vi "MENU.vi"() -> ()   [LabVIEW 2019]
panel:
  in  "Tab Control":T1(tab)
  out "DAC 2":dbl
  out "DAC 1":dbl
  in  "ADC 1 control":dbl
  out "ADC 1":dbl(knob) caption="Gauge" scale=0.0..10.0
  in  "DAC 1":dbl(knob) caption="Gauge" scale=0.0..10.0
  out "DI7":bool
  out "DI8":bool
  out "DI9":bool
  out "DI10":bool
  in  "DI7":bool
  in  "DI8":bool
  in  "DI9":bool
  in  "DI10":bool
  in  "DI11":bool
  in  "DI12":bool
  in  "DI13":bool
  out "DI11":bool
  out "DI12":bool
  out "DI13":bool
  in  "DO2 2":bool
  in  "DO3 2":bool
  in  "DO4 2":bool
  out "DO2":bool
  out "DO3":bool
  out "DO4":bool
  in  "DO5 2":bool
  in  "DO6 2":bool
  out "DO5":bool
  out "DO6":bool
  in  "DAC 2":dbl(knob) caption="Gauge" scale=0.0..10.0
  in  "PRODUCCION":bool
  in  "MANUAL":bool
  in  "I/O´S":bool
  in  "ESTADISTICAS":bool
  in  "PRINCIPAL":bool
  in  "stop":bool
  # "BIENVENIDO A LA MAQUINA MKI"
  # "SISTEMA DE PRODUCCIÓN"
  # "ESTADISTICAS DE PRODUCCIÓN"
  # "MONITOR DE ENTRAD Y SALIDAS"
  # "SISTEMA DE CONTROL MANUAL"
  # "ANALOGICO"
  # "SALIDAS"
  # "ENTRADAS"
  # "BYPASS"
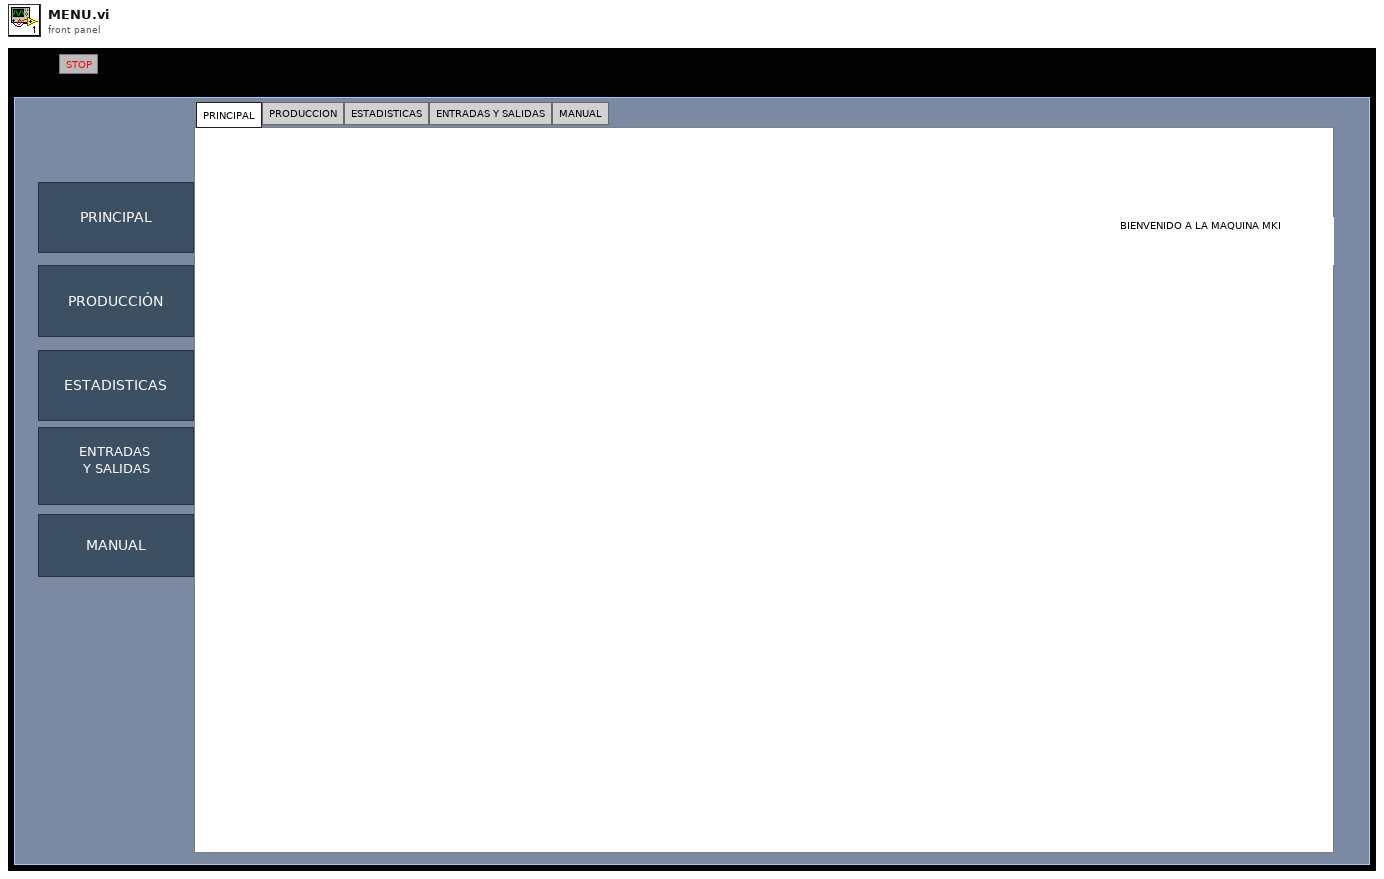
[diagram p1: front panel]
types:
  T1 = enum32{"PRINCIPAL", "PRODUCCION", "ESTADISTICAS", "ENTRADAS Y SALIDAS", "MANUAL"}
  T2 = enum32{"PRINCIPAL", "PPRODUCCION", "ESTADISTICAS", "ENTRADAS Y SALIDAS", "MANUAL"}
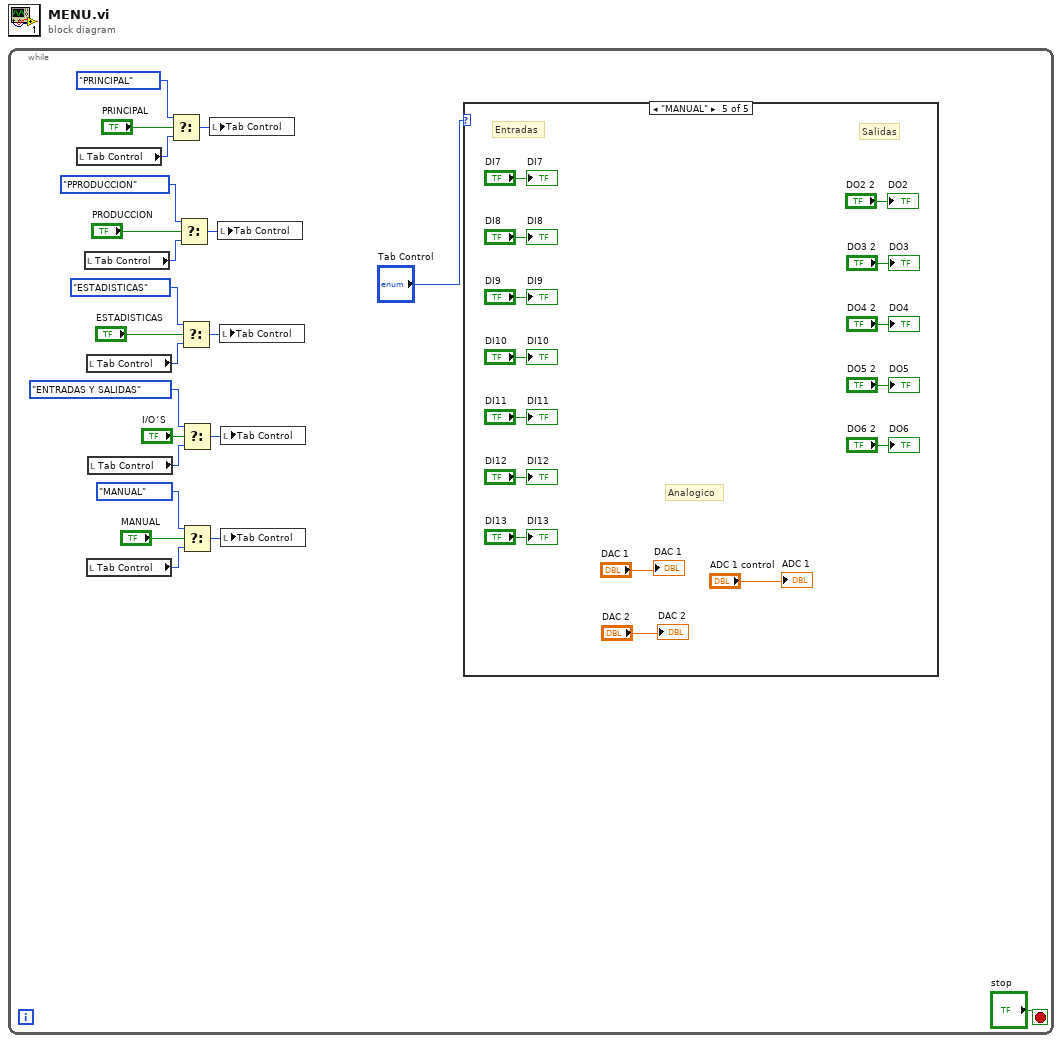
[diagram p0: block diagram]
diagram:
  n1 = while {
    stop <- "stop" stop-if-true
    n2 = local read "Tab Control"() -> (w21:T1)
    n3 = local read "Tab Control"() -> (w18:T1)
    n4 = local read "Tab Control"() -> (w15:T1)
    n5 = local read "Tab Control"() -> (w12:T1)
    n6 = local read "Tab Control"() -> (w9:T1)
    n7 = Select(t=T2."PRINCIPAL" ("Tab Control"), s="PRINCIPAL", f=w21) -> (s? t:f=w20:u32)
    n8 = Select(t=T2."PPRODUCCION" ("Tab Control"), s="PRODUCCION", f=w18) -> (s? t:f=w19:u32)
    n9 = Select(t=T2."ESTADISTICAS" ("Tab Control"), s="ESTADISTICAS", f=w15) -> (s? t:f=w14:u32)
    n10 = Select(t=T2."ENTRADAS Y SALIDAS" ("Tab Control"), s="I/O´S", f=w9) -> (s? t:f=w8:u32)
    n11 = Select(t=T2."MANUAL" ("Tab Control"), s="MANUAL", f=w12) -> (s? t:f=w13:u32)
    n12 = local write "Tab Control"(w20) -> ()
    n13 = local write "Tab Control"(w19) -> ()
    n14 = local write "Tab Control"(w14) -> ()
    n15 = local write "Tab Control"(w8) -> ()
    n16 = local write "Tab Control"(w13) -> ()
    n17 = case shown="\"MANUAL\"" "Tab Control" {
      frame "PRINCIPAL", Default {
      }
      frame "PRODUCCION" {
      }
      frame "ESTADISTICAS" {
      }
      frame "ENTRADAS Y SALIDAS" {
      }
      frame "MANUAL" {
        # "Analogico"
        # "Salidas"
        # "Entradas"
        "DI7" <- "DI7"
        "DO2" <- "DO2 2"
        "DO3" <- "DO3 2"
        "DO4" <- "DO4 2"
        "DO5" <- "DO5 2"
        "DO6" <- "DO6 2"
        "DI8" <- "DI8"
        "DI9" <- "DI9"
        "DI10" <- "DI10"
        "DI11" <- "DI11"
        "DI12" <- "DI12"
        "DI13" <- "DI13"
        "ADC 1" <- "ADC 1 control"
        "DAC 1" <- "DAC 1"
        "DAC 2" <- "DAC 2"
      }
    }
  }
